vi "AddSameKeys_ThrowExpectedError.vi"(8 "error in (no error)":errorcluster) -> (0 "error out":errorcluster)   [LabVIEW 2013]
uses:
  DictionaryStringClass/DictionaryString.lvclass
  <vilib>/addons/_JKI Toolkits/Caraya/classes/Assert/Assert.lvclass
  <vilib>/addons/_JKI Toolkits/Caraya/classes/Test/Test.lvclass
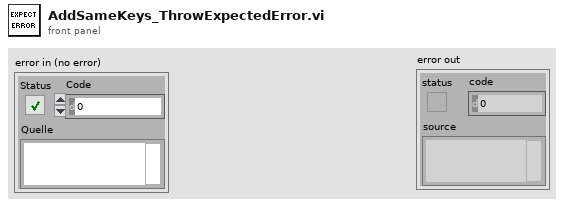
[diagram p1: front panel]
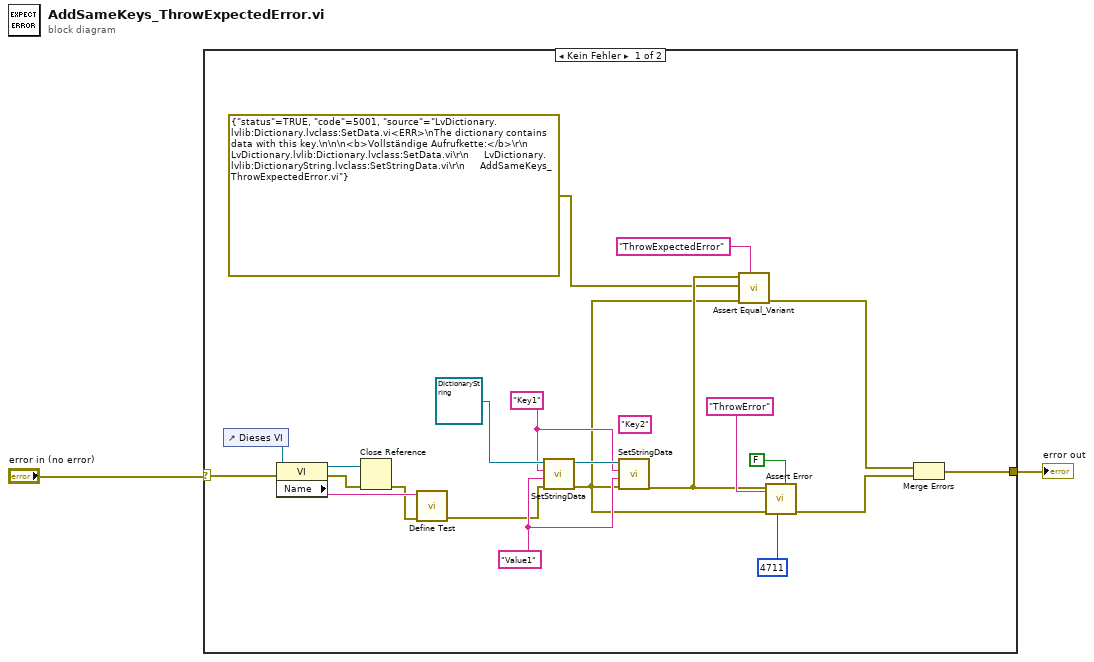
[diagram p0: block diagram]
diagram:
  n1 = case shown="Kein Fehler" "error in (no error)" {
    selector: "error in (no error)" -> [w17 w24]
    tunnel: [w5 w24] -> w2
    frame No Error {
      (unwired) "Key2" ("Name")
      w21 = "Value1" ("Value")
      w10 = "Key1" ("Name")
      n2 = control-ref of="Dieses VI"() -> (w19:refnum<vi>)
      n3 = property class="VI"(reference=w19, error in=w17) -> (reference out=w16:refnum<vi>, error out=w15:errorcluster, "Name"=w18:string)
      n4 = Close Reference(reference=w16, error in (no error)=w15) -> (error out=w13:errorcluster)
      n5 = call <vilib>:"Define Test.vi"("error in (no error)"=w13, "Label (VI Title)"=w18) -> ("error out"=w12:errorcluster)  [unwired: 9 in]
      n6 = call-dynamic "SetStringData.vi"("error in (no error)"=w12, "Value"=w21, "Name"=w10, "DictionaryString Eingang"=refnum<class "DictionaryString.lvclass"> refnum ("LvDictionary.lvlib:DictionaryString.lvclass")) -> ("error out"=w8:errorcluster, "DictionaryString Ausgang"=w22:refnum<class "DictionaryString.lvclass">)  [unwired: 6 in]
      n7 = call-dynamic "SetStringData.vi"("error in (no error)"=w8, "Value"=w21, "Name"=w10, "DictionaryString Eingang"=w22) -> ("error out"=w9:errorcluster)  [unwired: 6 in, 1 out]
      n8 = call <vilib>:"Assert Equal_Variant.vi"("Label"="ThrowExpectedError", "error in (no error)"=w8, "Y"=errorcluster {"status"=TRUE, "code"=5001, "source"="LvDictionary.lvlib:Dictionary.lvclass:SetData.vi<ERR>\nThe dictionary contains data with this key.\n\n\n<b>Vollständige Aufrufkette:</b>\r\n     LvDictionary.lvlib:Dictionary.lvclass:SetData.vi\r\n     LvDictionary.lvlib:DictionaryString.lvclass:SetStringData.vi\r\n     AddSameKeys_ThrowExpectedError.vi"} ("error out"), "X"=w9) -> ("error out"=w4:errorcluster)  [unwired: 7 in]
      n9 = call <vilib>:"Assert Error.vi"("Assert Only? (F)"=FALSE, "error code (1)"=4711, "Label"="ThrowError", "error in (no error)"=w8, "Error?"=w9) -> ("error out"=w6:errorcluster)  [unwired: 6 in]
      n10 = Merge Errors(w4, w6) -> (w5:errorcluster)
    }
    frame Error {
    }
  }
  "error out" <- w2
